vi "converter.vi"() -> ()   [LabVIEW 2017]
panel:
  in  "Radio Buttons":enum32{"Oct", "Dec", "Hex"}(ring)
  out "String":string
  in  "stop":bool
  out "Array 2":bool[](array[boolean])
  in  "Array":bool[](array[boolean])
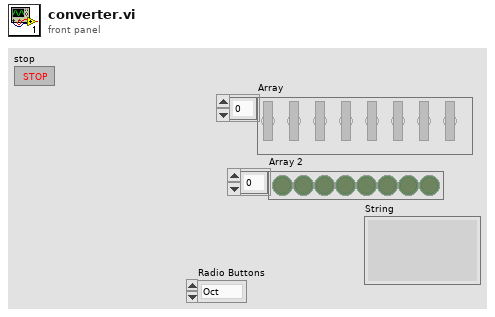
[diagram p1: front panel]
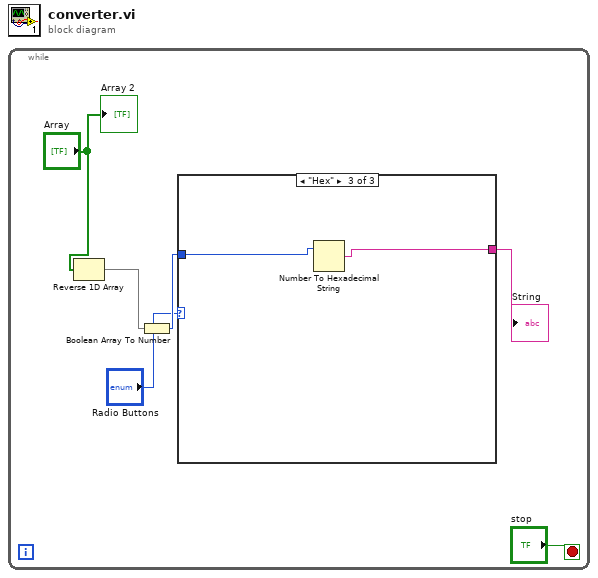
[diagram p0: block diagram]
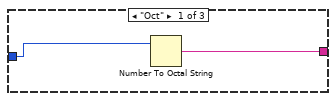
[diagram p2: hidden frame]
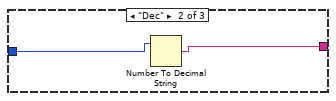
[diagram p3: hidden frame]
diagram:
  n1 = while {
    stop <- "stop" stop-if-true
    n2 = Reverse 1D Array(array="Array") -> (reversed array=w1:bool[])
    n3 = Boolean Array To Number(Boolean array=w1) -> (number=w5:u32)
    n4 = case shown="\"Hex\"" "Radio Buttons" {
      tunnel: w5 -> [w8 w10 w12]
      tunnel: [w7 w9 w11] -> w4
      frame "Oct" {
        n5 = Number To Octal String(2:w8) -> (0:w7:string)  [unwired: 1 in]
      }
      frame "Dec" {
        n6 = Number To Decimal String(number=w10) -> (decimal integer string=w9:string)  [unwired: 1 in]
      }
      frame "Hex" {
        n7 = Number To Hexadecimal String(2:w12) -> (0:w11:string)  [unwired: 1 in]
      }
    }
    "String" <- w4
    "Array 2" <- "Array"
  }
